vi "Receive Batch Node Actors VI Ref.vi"(6 "Paras In":variant, 7 "Actors In":refnum<class "System Actor.lvclass">[](array[class]), 8 "error in (no error)":errorcluster, 10 "VI Refs In":refnum<vi>[](array[refnum]), 11 "Simple Numeric Map Node Controller in":refnum<class "Simple Numeric Map Node Controller.lvclass">) -> (0 "error out":errorcluster, 3 "Simple Numeric Map Node Controller out":refnum<class "Simple Numeric Map Node Controller.lvclass">, 5 "Actors Out":refnum<class "System Actor.lvclass">[](array[class]))   [LabVIEW 2024, in "Simple Numeric Map Node Controller.lvclass"]
uses:
  Simple Numeric Map Node Controller.lvclass
  Ancestor Class/Messenger/Mail Strategy/Mail Strategy.lvclass
  Ancestor Class/Actor/System Actor/System Actor.lvclass
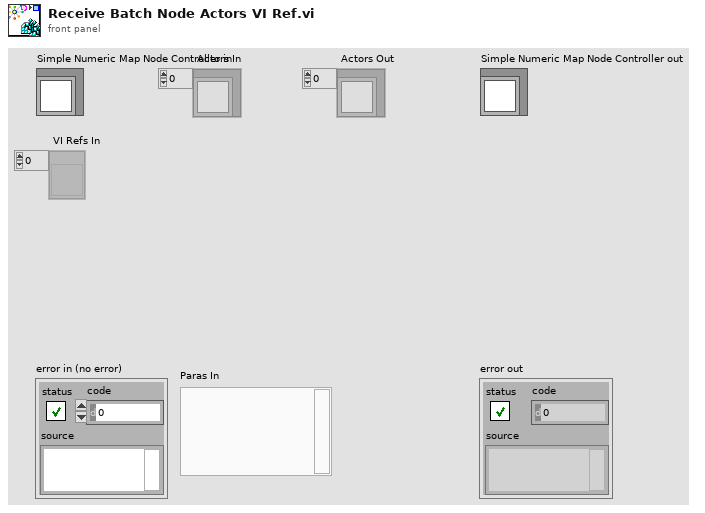
[diagram p1: front panel]
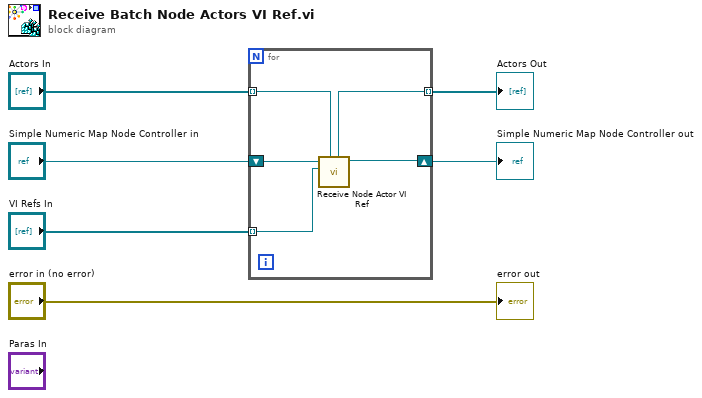
[diagram p0: block diagram]
diagram:
  n1 = for {
    tunnel: "Actors In" -> [w11] mode=indexing
    tunnel: [w10] -> w5 mode=indexing
    shift-right: [w8] -> w3
    shift-left: "Simple Numeric Map Node Controller in" -> [w9]
    tunnel: "VI Refs In" -> [w7] mode=indexing
    n2 = call-dynamic "Receive Node Actor VI Ref.vi"("System Actor In"=w11, "VI Refnum"=w7, "Simple Numeric Map Node Controller in"=w9) -> ("Simple Numeric Map Node Controller out"=w8:refnum<class "Simple Numeric Map Node Controller.lvclass">, "System Actor Out"=w10:refnum<class "System Actor.lvclass">)  [unwired: 6 in, 1 out]
  }
  "Simple Numeric Map Node Controller out" <- w3
  "Actors Out" <- w5
  "error out" <- "error in (no error)"
